vi "Event-Trigger-mode.vi"(7 "Trigger mode":T1, 8 "error in (no error)":errorcluster, 10 "Data ref. in":refnum<data-value>, 11 "UI ref. in":refnum<data-value>) -> (0 "error out":errorcluster, 2 "Data ref.":refnum<data-value>, 3 "UI ref.":refnum<data-value>)   [LabVIEW 2013, in "CameraVision.lvlib" / "CV-UI.lvclass"]
uses:
  CV-UI.lvclass
  Main/CV-Main.lvclass
  Main/Acquisition/Trigger-modes.ctl
  Control-names.ctl
  Main/Acquisition/CV-Acquisition.lvclass
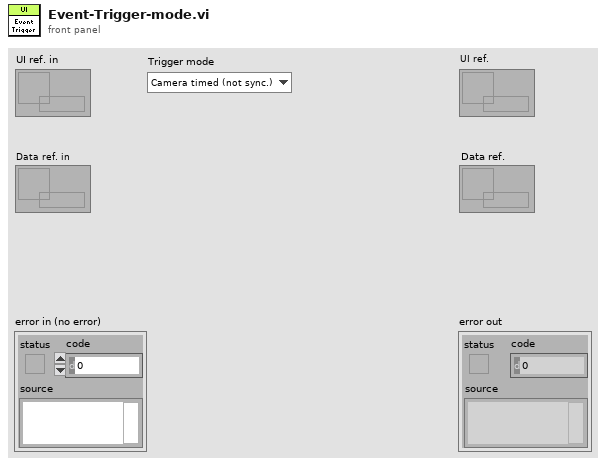
[diagram p1: front panel]
types:
  T1 = typedef "CameraVision.lvlib/CV-Acquisition.lvclass/Trigger-modes.ctl" = enum16{"Camera timed (not sync.)", "Framegrabber timed (sync.)", "Software timed (sync.)", "External timing (sync.)", "Manual (sync.)", "Gated - camera (not sync.)", "Gated - grabber (sync.)", "Gated - software (sync.)", "Gated - external (sync.)"}
  T2 = typedef "CameraVision.lvlib/CV-UI.lvclass/Control-names.ctl" = enum16{"Start acquisition", "Activate", "Stop acquisition", "Settings type", "Load settings", "Save settings", "Import images", "Camera selector", "Image type selector", "Batch browser", "Image refresh", "Parameter tabs", "Displays", "Processing tabs", "Processing selector", "Map characteristic", "Show info", "Manual trigger"}
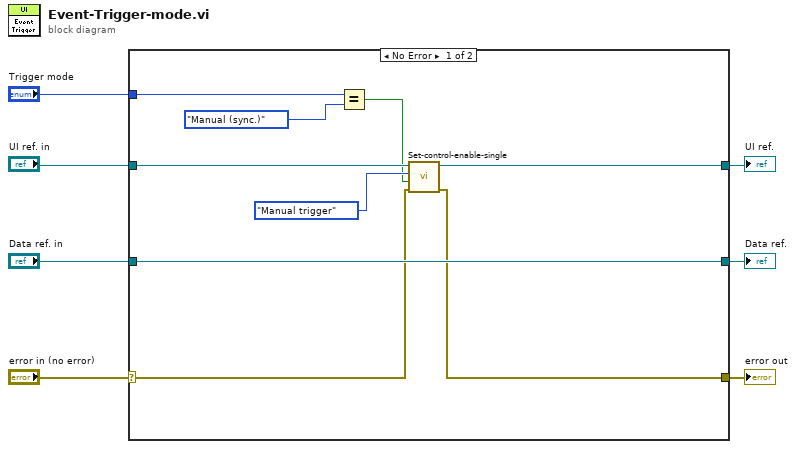
[diagram p0: block diagram]
diagram:
  n1 = case shown="No Error" "error in (no error)" {
    selector: "error in (no error)" -> [w11 w19]
    tunnel: [w10 w19] -> w6
    tunnel: [w8 w18] -> w4
    tunnel: "UI ref. in" -> [w13 w18]
    tunnel: "Data ref. in" -> [w16 w17]
    tunnel: "Trigger mode" -> [w15 _]
    tunnel: [w16 w17] -> w1
    frame No Error {
      n2 = Equal?(x=w15, y=Trigger-modes."Manual (sync.)") -> (x = y?=w9:bool)
      n3 = call "Set-control-enable-single.vi"("error in (no error)"=w11, "Enable?"=w9, "Control name"=Control-names."Manual trigger" ("Control"), "UI ref. in"=w13) -> ("error out"=w10:errorcluster, "UI ref."=w8:refnum<data-value>)  [unwired: 6 in]
    }
    frame Error {
    }
  }
  "error out" <- w6
  "Data ref." <- w1
  "UI ref." <- w4
